vi "Balance.vi"(8 "error in (no error)":errorcluster, 11 "CR5 in":refnum<class "CR5.lvclass">) -> (0 "error out":errorcluster, 3 "CR5 out":refnum<class "CR5.lvclass">)   [LabVIEW 2019, in "CR5.lvclass"]
uses:
  CR5.lvclass
  Reusable/Session APIs/Serial/Serial Session.lvclass
  CR5.lvclass/CR5.ctl
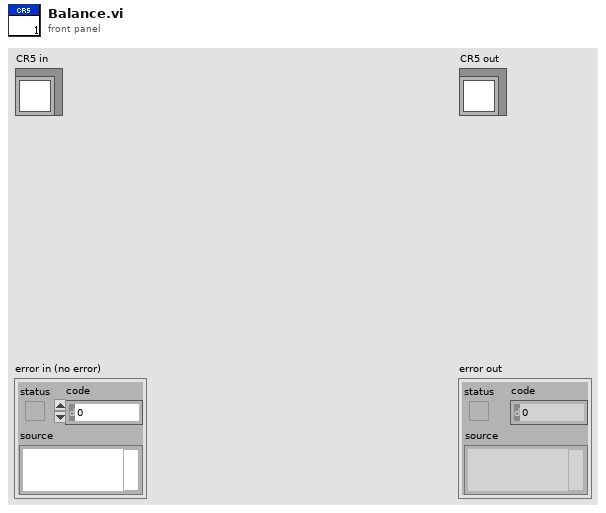
[diagram p1: front panel]
types:
  T1 = typedef "Session - Root.lvclass/Session Handle.ctl" = refnum<data-value>
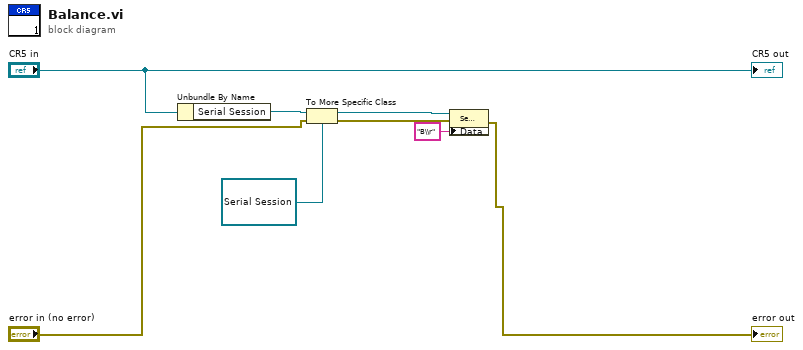
[diagram p0: block diagram]
diagram:
  n1 = Unbundle By Name("CR5 in") -> ("Serial Session"=w8:T1)
  n2 = To More Specific Class(target class=refnum<data-value> refnum, reference=w8, error in="error in (no error)") -> (specific class reference=w5:refnum<data-value>, error out=w6:errorcluster)
  n3 = property class="Serial Session"(reference=w5, error in=w6, "Data"="B\\r") -> (error out=→"error out":errorcluster)  [unwired: 1 out]
  "CR5 out" <- "CR5 in"
